vi "Is Empty234.vi"(11 "MsgPackMap in":refnum<class "MsgPackMap.lvclass">) -> (3 "MsgPackMap out":refnum<class "MsgPackMap.lvclass">)   [LabVIEW 2020]
uses:
  MsgPackMap.lvclass/MsgPackMap.ctl
  MsgPackMap.lvclass
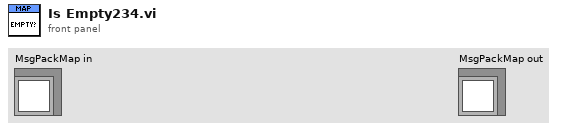
[diagram p1: front panel]
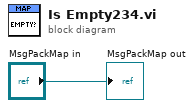
[diagram p0: block diagram]
diagram:
  "MsgPackMap out" <- "MsgPackMap in"
